vi "脉冲脚本.vi"(4 "4-wire":bool, 6 "脉冲":T1 {"测试参数"."反向极限电流(mA)" min=0.0 max=3000.0; "测试参数"."反向电压(V)" min=-40.0 max=40.0; "测试参数"."读取电压(V)" min=-40.0 max=40.0; "测试参数"."正向极限电流(mA)" min=0.0 max=3000.0; "测试参数"."正向电压(V)" min=-40.0 max=40.0}, 8 "错误输入（无错误）":errorcluster, 11 "方向(T:正向)":bool=TRUE) -> (0 "错误输出":errorcluster, 1 "Script":string)   [LabVIEW 2020, in "功能选择.xctl"]
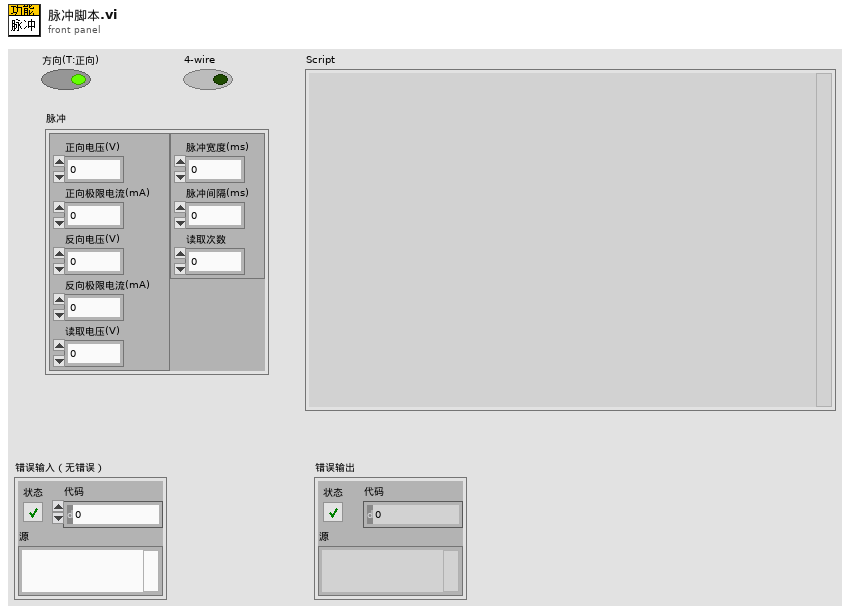
[diagram p1: front panel]
types:
  T1 = typedef "功能选择.xctl/脉冲参数.ctl" = cluster{"测试参数":cluster{"正向电压(V)":dbl, "正向极限电流(mA)":dbl, "反向电压(V)":dbl, "反向极限电流(mA)":dbl, "读取电压(V)":dbl}, "时序参数":cluster{"脉冲宽度(ms)":dbl, "脉冲间隔(ms)":dbl, "读取次数":u32}}
  T2 = cluster{"正向电压(V)":dbl, "正向极限电流(mA)":dbl, "反向电压(V)":dbl, "反向极限电流(mA)":dbl, "读取电压(V)":dbl}
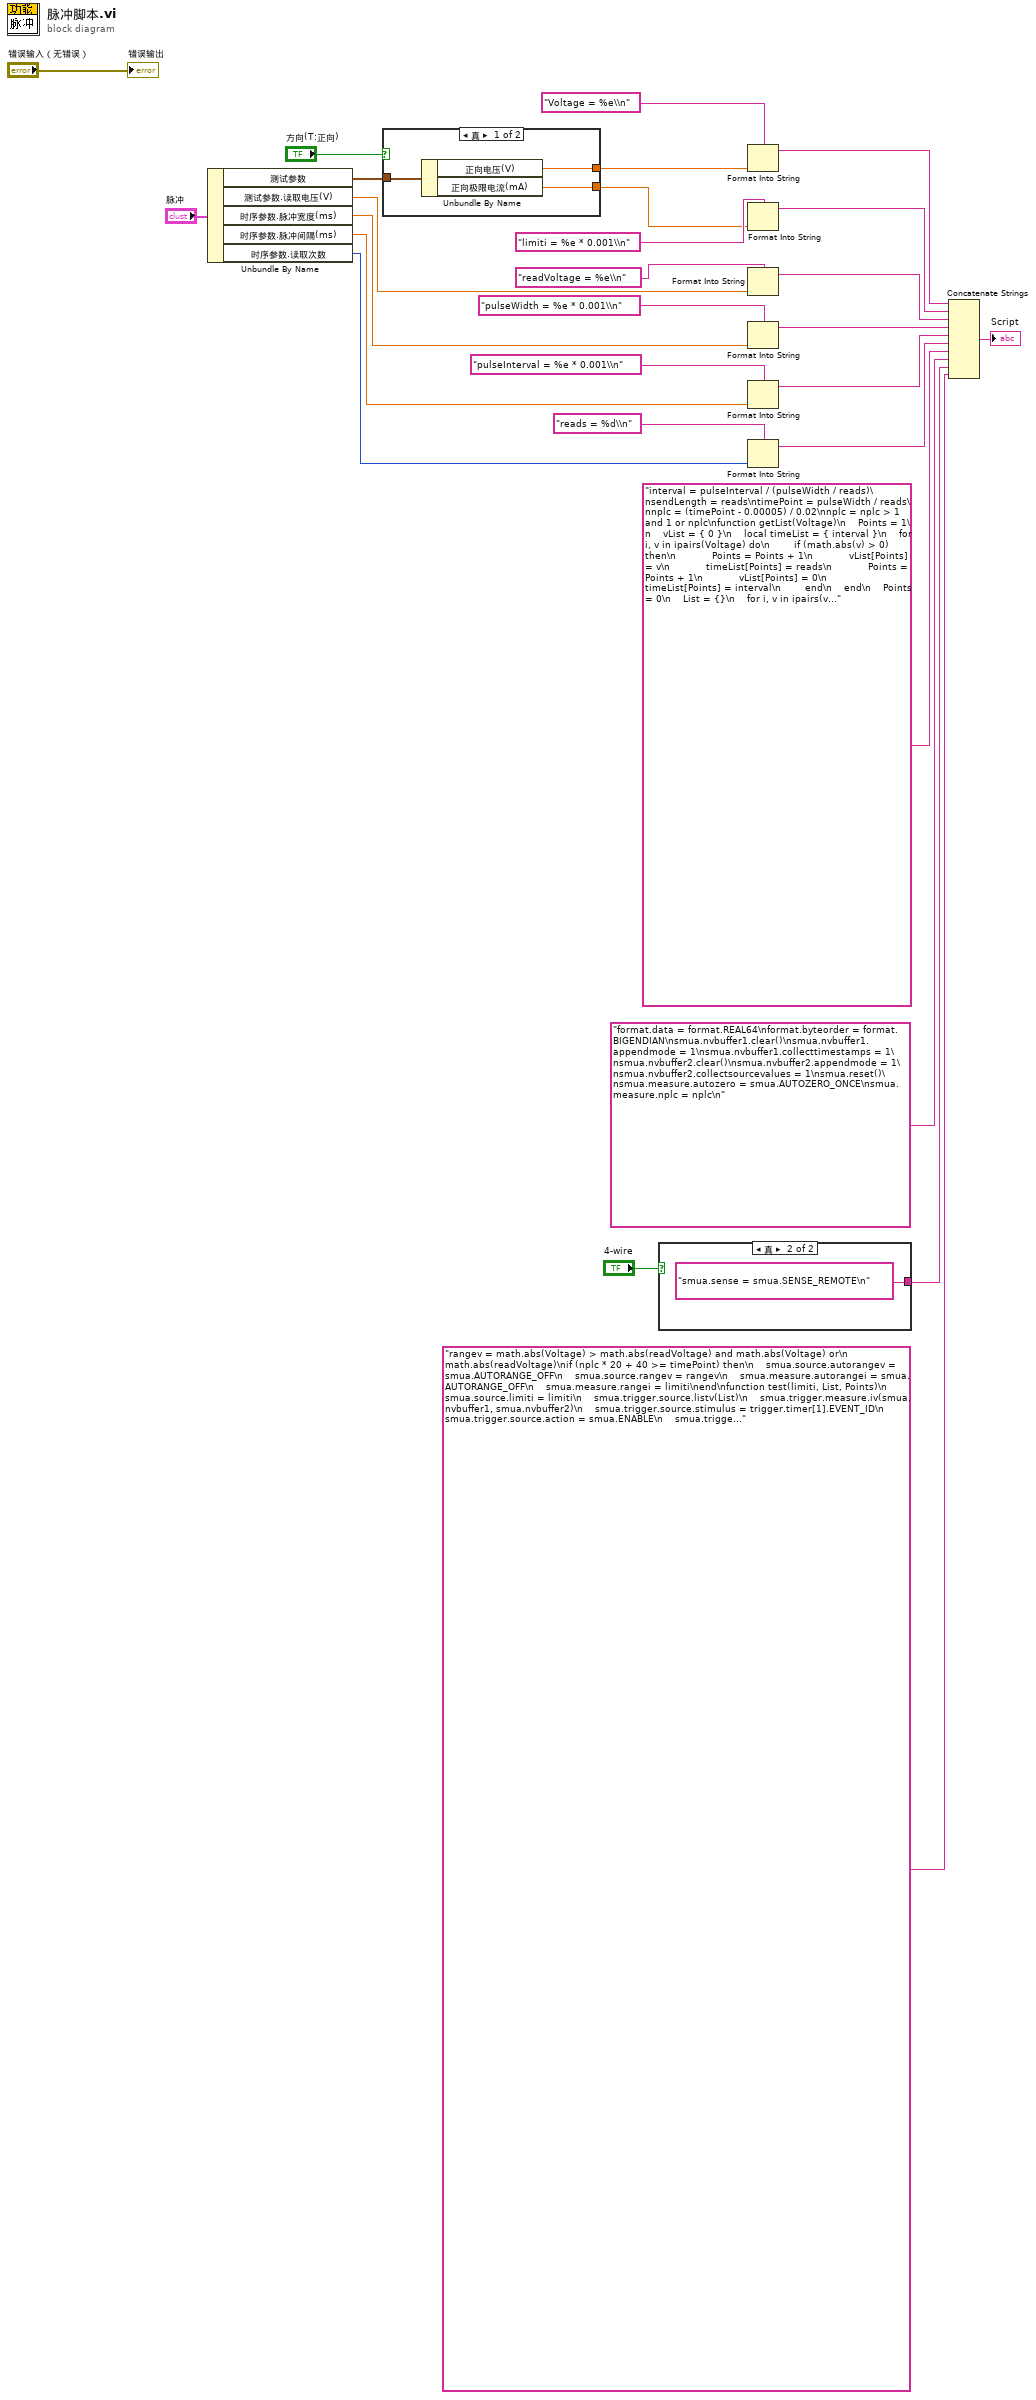
[diagram p0: block diagram]
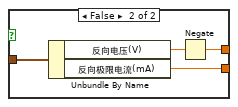
[diagram p2: hidden frame]
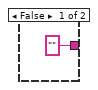
[diagram p3: hidden frame]
diagram:
  n1 = Unbundle By Name("脉冲") -> ("测试参数"=w12:T2, "测试参数.读取电压(V)"=w7:dbl, "时序参数.脉冲宽度(ms)"=w9:dbl, "时序参数.脉冲间隔(ms)"=w1:dbl, "时序参数.读取次数"=w8:u32)
  n2 = case shown="真" "方向(T:正向)" {
    tunnel: w12 -> [w31 w35]
    tunnel: [w30 w32] -> w14
    tunnel: [w29 w34] -> w13
    frame True {
      n3 = Unbundle By Name(w31) -> ("正向电压(V)"=w30:dbl, "正向极限电流(mA)"=w29:dbl)
    }
    frame False {
      n4 = Unbundle By Name(w35) -> ("反向电压(V)"=w33:dbl, "反向极限电流(mA)"=w34:dbl)
      n5 = Negate(x=w33) -> (-x=w32:dbl)
    }
  }
  n6 = case shown="真" "4-wire" {
    tunnel: ["" "smua.sense = smua.SENSE_REMOTE\n"] -> w21
    frame False {
    }
    frame True {
    }
  }
  n7 = Format Into String(format string="Voltage = %e\\n" ("格式字符串"), w14) -> (resulting string=w25:string)  [unwired: 2 in, 1 out]
  n8 = Format Into String(format string="limiti = %e * 0.001\\n" ("格式字符串"), w13) -> (resulting string=w16:string)  [unwired: 2 in, 1 out]
  n9 = Format Into String(format string="readVoltage = %e\\n" ("格式字符串"), w7) -> (resulting string=w15:string)  [unwired: 2 in, 1 out]
  n10 = Format Into String(format string="pulseWidth = %e * 0.001\\n", w9) -> (resulting string=w10:string)  [unwired: 2 in, 1 out]
  n11 = Format Into String(format string="pulseInterval = %e * 0.001\\n", w1) -> (resulting string=w2:string)  [unwired: 2 in, 1 out]
  n12 = Format Into String(format string="reads = %d\\n" ("格式字符串"), w8) -> (resulting string=w5:string)  [unwired: 2 in, 1 out]
  n13 = Concatenate Strings(w25, w16, w15, w10, w2, w5, "interval = pulseInterval / (pulseWidth / reads)\nsendLength = reads\ntimePoint = pulseWidth / reads\nnplc = (timePoint - 0.00005) / 0.02\nnplc = nplc > 1 and 1 or nplc\nfunction getList(Voltage)\n    Points = 1\n    vList = { 0 }\n    local timeList = { interval }\n    for i, v in ipairs(Voltage) do\n        if (math.abs(v) > 0) then\n            Points = Points + 1\n            vList[Points] = v\n            timeList[Points] = reads\n            Points = Points + 1\n            vList[Points] = 0\n            timeList[Points] = interval\n        end\n    end\n    Points = 0\n    List = {}\n    for i, v in ipairs(vList) do\n        for i = 1, timeList[i] do\n            Points = Points + 1\n            List[Points] = v\n        end\n    end\n    return List, Points\nend\nList, Points = getList({ Voltage, readVoltage })\n" ("字符串"), "format.data = format.REAL64\nformat.byteorder = format.BIGENDIAN\nsmua.nvbuffer1.clear()\nsmua.nvbuffer1.appendmode = 1\nsmua.nvbuffer1.collecttimestamps = 1\nsmua.nvbuffer2.clear()\nsmua.nvbuffer2.appendmode = 1\nsmua.nvbuffer2.collectsourcevalues = 1\nsmua.reset()\nsmua.measure.autozero = smua.AUTOZERO_ONCE\nsmua.measure.nplc = nplc\n", w21, "rangev = math.abs(Voltage) > math.abs(readVoltage) and math.abs(Voltage) or\n             math.abs(readVoltage)\nif (nplc * 20 + 40 >= timePoint) then\n    smua.source.autorangev = smua.AUTORANGE_OFF\n    smua.source.rangev = rangev\n    smua.measure.autorangei = smua.AUTORANGE_OFF\n    smua.measure.rangei = limiti\nend\nfunction test(limiti, List, Points)\n    smua.source.limiti = limiti\n    smua.trigger.source.listv(List)\n    smua.trigger.measure.iv(smua.nvbuffer1, smua.nvbuffer2)\n    smua.trigger.source.stimulus = trigger.timer[1].EVENT_ID\n    smua.trigger.source.action = smua.ENABLE\n    smua.trigger.measure.action = smua.ENABLE\n    smua.trigger.count = Points\n    smua.trigger.arm.stimulus = trigger.EVENT_ID\n    trigger.timer[1].reset()\n    trigger.timer[1].stimulus = smua.trigger.ARMED_EVENT_ID\n    trigger.timer[1].passthrough = false\n    trigger.timer[1].delay = timePoint\n    trigger.timer[1].count = Points\n    smua.trigger.initiate()\n    smua.trigger.arm.set()\nend\nfunction sendData()\n    repeat\n        if (bit.test(status.operation.instrument.smua.condition, 4) == false) then\n            return\n        elseif (smua.nvbuffer1.n > Stop) then\n            print(\"{\" .. sendLength .. \"}\")\n            printbuffer(Start, Stop, smua.nvbuffer1.timestamps)\n            printbuffer(Start, Stop, smua.nvbuffer2.sourcevalues)\n            printbuffer(Start, Stop, smua.nvbuffer1)\n            printbuffer(Start, Stop, smua.nvbuffer2)\n            Start = Start + sendLength\n            Stop = Stop + sendLength\n        end\n        delay(timePoint)\n    until (false)\nend\nfunction sendLastData()\n    Stop = smua.nvbuffer1.n\n    print(\"{\" .. Stop - Start + 1 .. \"}\")\n    printbuffer(Start, Stop, smua.nvbuffer1.timestamps)\n    printbuffer(Start, Stop, smua.nvbuffer2.sourcevalues)\n    printbuffer(Start, Stop, smua.nvbuffer1)\n    printbuffer(Start, Stop, smua.nvbuffer2)\n    print(\"{done}\")\nend\nif (Points > 0) then\n    Start = 1\n    Stop = sendLength\n    smua.source.output = smua.OUTPUT_ON\n    test(limiti, List, Points)\n    sendData()\n    smua.source.output = smua.OUTPUT_OFF\n    sendLastData()\nelse\n    print(\"{done}\")\nend\nreset()") -> (→"Script":string)
  "错误输出" <- "错误输入（无错误）"
